vi "Main.vi"() -> ()   [LabVIEW 2021]
uses:
  Direction.ctl
  Coordinates.ctl
  Game Board_class/Game Board.lvclass
  Fruit_class/Fruit.lvclass
  Snake_class/Snake.lvclass
panel:
  out "Score":u32
  out "Board":u32[][](array[colorbox])
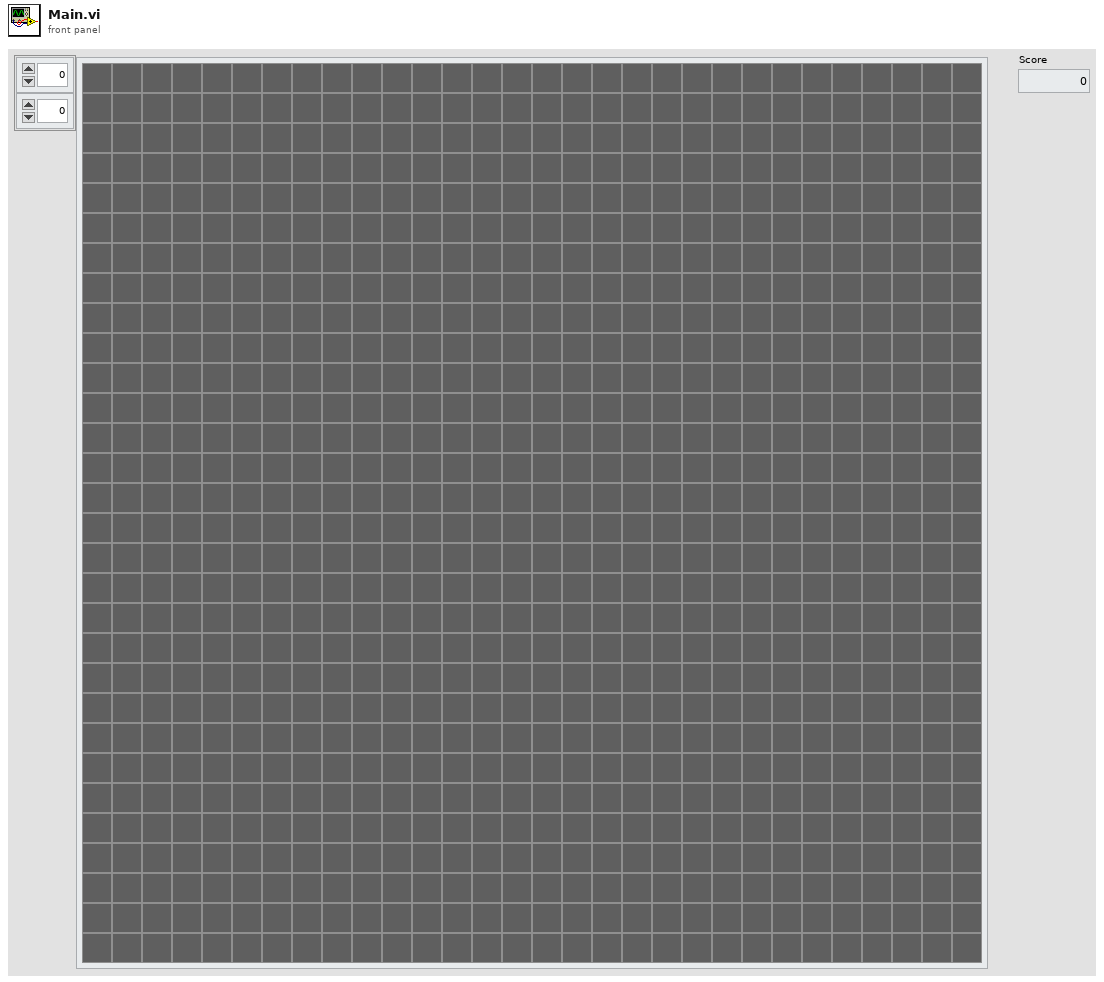
[diagram p1: front panel]
types:
  T1 = typedef "Coordinates.ctl" = cluster{"X":i32, "Y":i32}
  T2 = typedef "Direction.ctl" = enum16{"up", "down", "left", "right"}
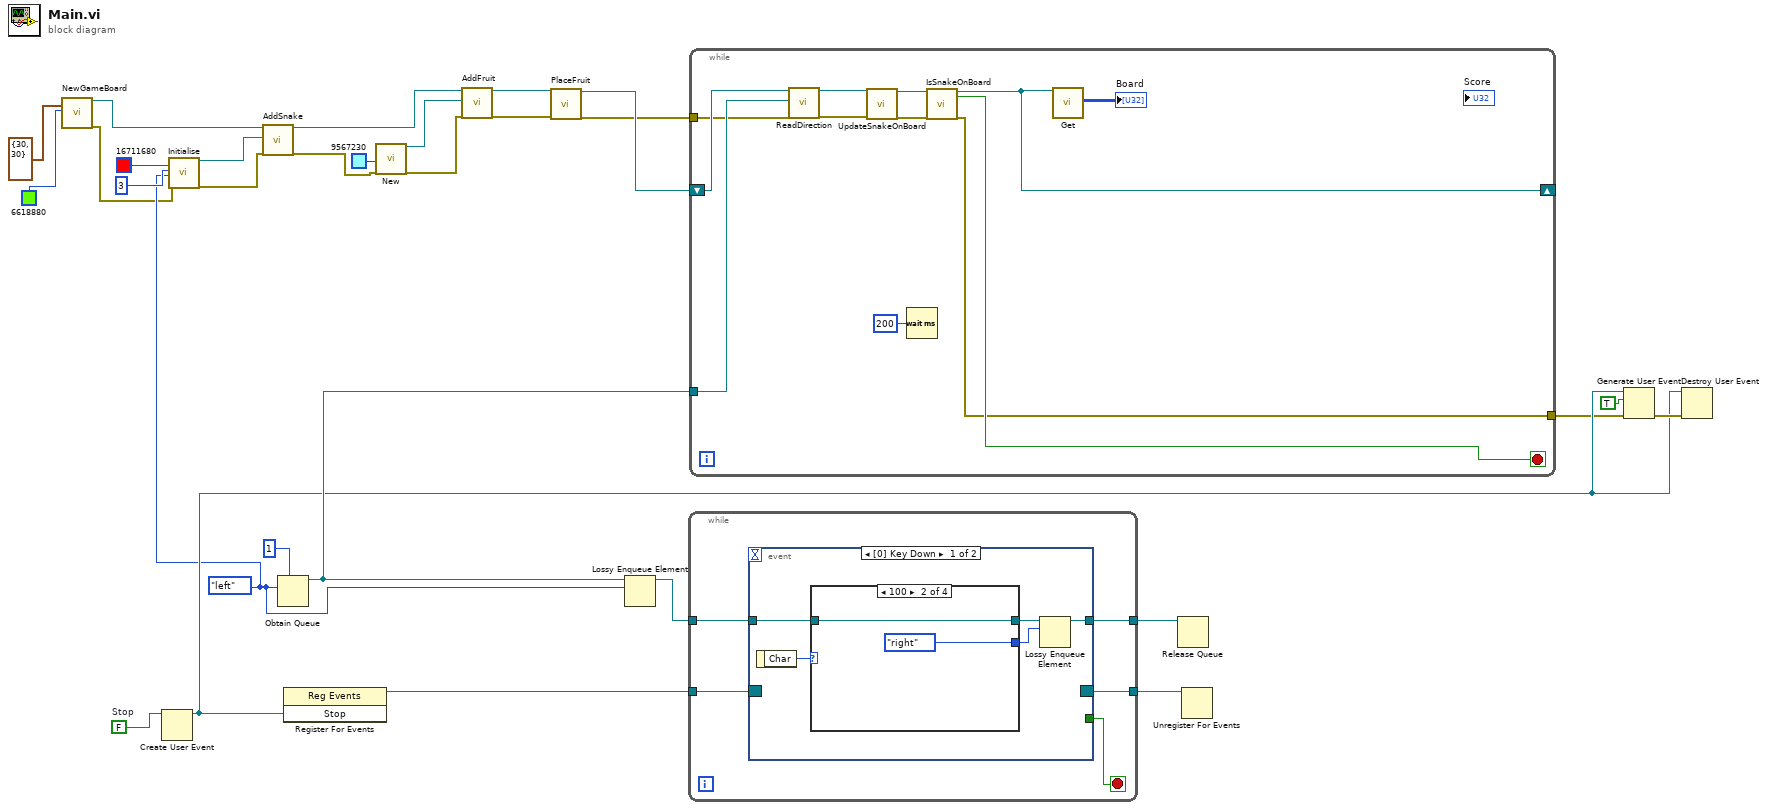
[diagram p0: block diagram]
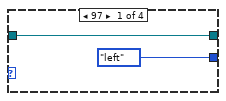
[diagram p2: hidden frame]
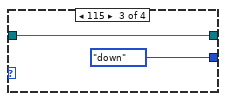
[diagram p3: hidden frame]
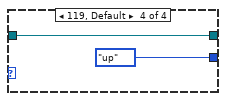
[diagram p4: hidden frame]
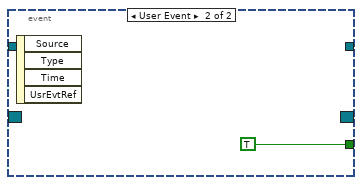
[diagram p5: hidden frame]
diagram:
  w20 = FALSE  # Stop
  w15 = Direction."left" ("Enum")
  n1 = call "NewGameBoard.vi"("Grid Size"=T1 {"X"=30, "Y"=30}, "Color Box"=u32 6618880) -> ("object out"=w13:refnum<class "Game Board.lvclass">, "error out"=w9:errorcluster)  [unwired: 16 in]
  n2 = Create User Event(user event datatype=w20) -> (user event=w23:refnum<user-event>)  [unwired: 1 in, 1 out]
  n3 = call "Initialise.vi"("Snake Colour"=u32 16711680, "Starting Elements"=3, "Direction"=w15, "error in (no error)"=w9) -> ("object out"=w14:refnum<class "Snake.lvclass">, "error out"=w8:errorcluster)  [unwired: 14 in]
  n4 = call-dynamic "AddSnake.vi"("object in"=w13, "Snake in"=w14, "error in (no error)"=w8) -> ("object out"=w11:refnum<class "Game Board.lvclass">, "error out"=w7:errorcluster)  [unwired: 15 in]
  n5 = Obtain Queue(max queue size (-1, unlimited)=1, element data type=w15) -> (queue out=w26:refnum<queue>)  [unwired: 3 in, 2 out]
  n6 = register-events(w23) -> (reference out=w24:refnum<event-registration>)  [unwired: 2 in, 1 out]
  n7 = call "New.vi"("Colour"=u32 9567230, "error in (no error)"=w7) -> ("object out"=w10:refnum<class "Fruit.lvclass">, "error out"=w6:errorcluster)  [unwired: 16 in]
  n8 = call-dynamic "AddFruit.vi"("object in"=w11, "Fruit"=w10, "error in (no error)"=w6) -> ("object out"=w5:refnum<class "Game Board.lvclass">, "error out"=w4:errorcluster)  [unwired: 15 in]
  n9 = call-dynamic "PlaceFruit.vi"("object in"=w5, "error in (no error)"=w4) -> ("object out"=w3:refnum<class "Game Board.lvclass">, "error out"=w2:errorcluster)  [unwired: 16 in]
  n10 = Lossy Enqueue Element(queue=w26, element=w15) -> (queue out=w28:refnum<queue>)  [unwired: 1 in, 3 out]
  n11 = while {
    tunnel: w28 -> [w34]
    tunnel: [w33] -> w27
    tunnel: w24 -> [w32]
    tunnel: [w31] -> w21
    stop <- w30 stop-if-true
    n12 = event shown="[0] Key Down" {
      selector: w32 -> [_ _]
      dyn-events: [_ _] -> w31
      timeout: _ -> [_ _]
      tunnel: w34 -> [w38 _]
      tunnel: [w35 _] -> w33
      tunnel: [_ TRUE] -> w30
      event Key Down {
        n13 = event-data() -> ("Char"=w39:i16)  [unwired: 1 in]
        n14 = case shown="100" w39 {
          tunnel: w38 -> [w40 w43 w44 w46]
          tunnel: [w40 w43 w44 w46] -> w37
          tunnel: [Direction."left" ("Enum") Direction."right" ("Enum") Direction."down" ("Enum") Direction."up" ("Enum")] -> w36
          frame 97 {
          }
          frame 100 {
          }
          frame 115 {
          }
          frame 119, Default {
          }
        }
        n15 = Lossy Enqueue Element(queue=w37, element=w36) -> (queue out=w35:refnum<queue>)  [unwired: 1 in, 3 out]
      }
      event User Event {
        n16 = event-data() -> ()  [unwired: 1 in, 4 out]
      }
    }
  }
  n17 = while {
    tunnel: w26 -> [w59]
    tunnel: w2 -> [w57]
    shift-right: [w52] -> _
    shift-left: w3 -> [w58]
    tunnel: [w49] -> w1
    stop <- w50 stop-if-true
    n18 = call-dynamic "ReadDirection.vi"("object in"=w58, "Direction SEQ"=w59, "error in (no error)"=w57) -> ("object out"=w56:refnum<class "Game Board.lvclass">, "error out"=w55:errorcluster)  [unwired: 15 in]
    n19 = call-dynamic "UpdateSnakeOnBoard.vi"("object in"=w56, "error in (no error)"=w55) -> ("object out"=w53:refnum<class "Game Board.lvclass">, "error out"=w51:errorcluster)  [unwired: 16 in]
    n20 = Wait (ms)(milliseconds to wait=u32 200) -> ()  [unwired: 1 out]
    n21 = call-dynamic "IsSnakeOnBoard.vi"("object in"=w53, "error in (no error)"=w51) -> ("object out"=w52:refnum<class "Game Board.lvclass">, "Fail"=w50:bool, "error out"=w49:errorcluster)  [unwired: 15 in]
    n22 = call-dynamic "Get.vi"("object in"=w52) -> ("Game Board"=→"Board":u32[][])  [unwired: 17 in, 1 out]
  }
  n23 = Release Queue(queue=w27) -> ()  [unwired: 2 in, 3 out]
  n24 = Unregister For Events(event registration refnum=w21) -> ()  [unwired: 1 in, 1 out]
  n25 = Generate User Event(user event=w23, event data cluster=TRUE ("event data"), error in=w1) -> (error out=w25:errorcluster)  [unwired: 1 in, 1 out]
  n26 = Destroy User Event(user event=w23, error in=w25) -> ()  [unwired: 1 out]
